vi "SPI Block Write Bytes Of Event.vi"(1 "TimeOutOfMs":i32, 4 "EventType":u8, 5 "EventPin":i32, 6 "BlockNum":i32, 7 "BlockSize":i32, 9 "pWriteData":u8, 10 "SPIIndex":i32, 11 "DevHandle":i32) -> (2 "function return":i32, 3 "pWriteData out":u8)   [LabVIEW 2010, in "usb2spi.lvlib"]
doc: "int WINAPI SPI_BlockWriteBytesOfEvent(int DevHandle,int SPIIndex,unsigned char *pWriteData,int BlockSize,int BlockNum,int EventPin,unsigned char EventType,int TimeOutOfMs);"
uses:
  usb2spi.lvlib
  USB2XXX.dll
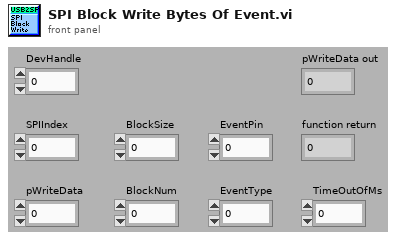
[diagram p1: front panel]
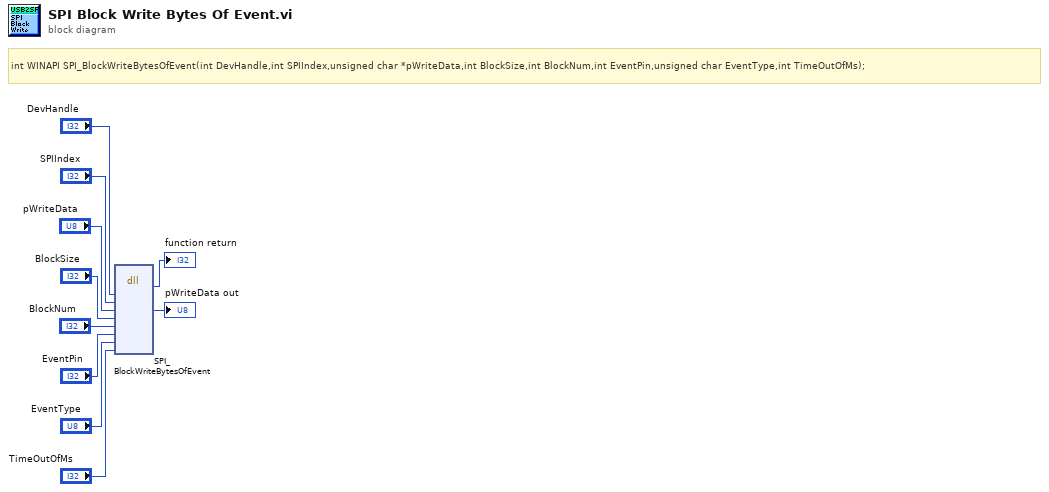
[diagram p0: block diagram]
diagram:
  # "int WINAPI SPI_BlockWriteBytesOfEvent(int DevHandle,int SPIIndex,unsigned char *pWriteData,int BlockSize,int BlockNum,int EventPin,unsigned char EventType,int TimeOutOfMs);"
  n1 = dll-call lib="G:/OtherWork/USB2XXX_Example/trunk/Labview/PublicFiles/usb2spi/USB2XXX.*" fn="SPI_BlockWriteBytesOfEvent"("DevHandle"="DevHandle", "SPIIndex"="SPIIndex", "pWriteData"="pWriteData", "BlockSize"="BlockSize", "BlockNum"="BlockNum", "EventPin"="EventPin", "EventType"="EventType", "TimeOutOfMs"="TimeOutOfMs") -> (→"function return":i32, "pWriteData"=→"pWriteData out":u8)  [unwired: 10 in, 2 out]
